vi "SQL表面型号删除.vi"(0 "Type_c":string, 11 "error in (no error)":errorcluster caption="错误输入（无错误）") -> (15 "error out":errorcluster caption="错误输出")   [LabVIEW 2017]
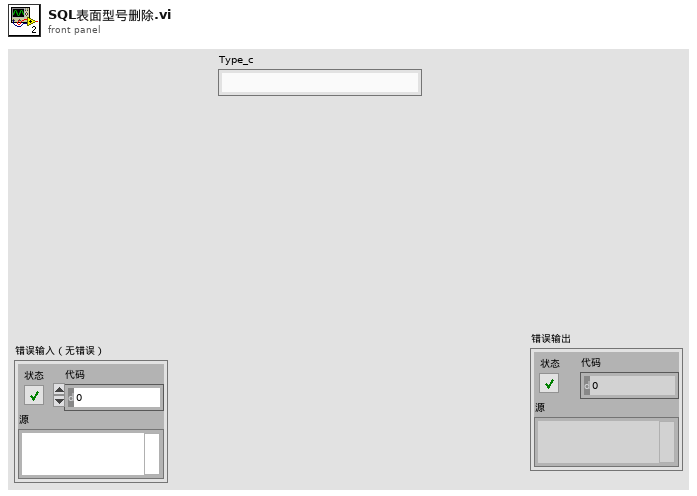
[diagram p1: front panel]
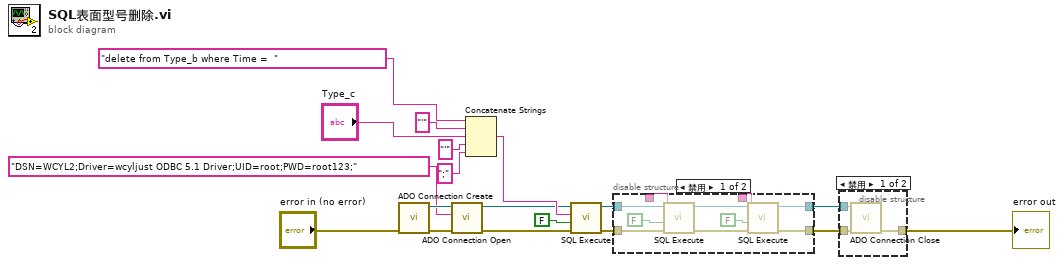
[diagram p0: block diagram]
diagram:
  n1 = call <userlib>:"ADO Connection Create.vi"("error in (no error)"="error in (no error)") -> ("error out"=w10:errorcluster, "ADODB._Connection Out"=w11:refnum<k7>)  [unwired: 9 in]
  n2 = call <userlib>:"ADO Connection Open.vi"("error in (no error)"=w10, "ConnectionString"="DSN=WCYL2;Driver=wcyljust ODBC 5.1 Driver;UID=root;PWD=root123;", "ADODB._Connection In"=w11) -> ("error out"=w5:errorcluster, "ADODB._Connection Out"=w6:refnum<k7>)  [unwired: 7 in]
  n3 = Concatenate Strings("delete from Type_b where Time =  " ("Command Text"), "'" ("字符串"), "Type_c", "'" ("字符串"), ";" ("字符串")) -> (w14:string)
  n4 = call <userlib>:"SQL Execute.vi"("error in (no error)"=w5, "Return Data (T)"=FALSE, "Command Text"=w14, "ADODB._Connection In"=w6) -> ("error out"=w4:errorcluster, "ADODB._Connection Out"=w1:refnum<k7>)  [unwired: 4 in, 2 out]
  n5 = disable-structure shown="禁用" {
    disable-tunnel: w4 -> [w26 w29]
    disable-tunnel: [w24 w29] -> w3
    disable-tunnel: [w23 w30] -> w2
    disable-tunnel: w1 -> [w21 w30]
    disable-tunnel: _ -> [w20 _]
    disable-tunnel: _ -> [w19 _]
    frame Disabled {
      n6 = call <userlib>:"SQL Execute.vi"("error in (no error)"=w26, "Return Data (T)"=FALSE, "Command Text"=w20, "ADODB._Connection In"=w21) -> ("error out"=w25:errorcluster, "ADODB._Connection Out"=w22:refnum<k7>)  [unwired: 4 in, 2 out]
      n7 = call <userlib>:"SQL Execute.vi"("error in (no error)"=w25, "Return Data (T)"=FALSE, "Command Text"=w19, "ADODB._Connection In"=w22) -> ("error out"=w24:errorcluster, "ADODB._Connection Out"=w23:refnum<k7>)  [unwired: 4 in, 2 out]
    }
    frame Enabled {
    }
  }
  n8 = disable-structure shown="禁用" {
    disable-tunnel: [w33 _] -> w8
    disable-tunnel: w3 -> [w32 _]
    disable-tunnel: w2 -> [w31 _]
    frame Disabled {
      n9 = call <userlib>:"ADO Connection Close.vi"("error in (no error)"=w32, "ADODB._Connection In"=w31) -> ("error out"=w33:errorcluster)  [unwired: 8 in, 1 out]
    }
    frame Enabled {
    }
  }
  "error out" <- w8
